vi "statusindicatorwithactivate.vi"(6 "String":string, 9 "Power":bool, 11 "Activate":bool) -> (0 "?":bool, 1 "?":bool, 2 "?":bool, 3 "?":bool, 4 "?":string)   [LabVIEW 2018, in "com.insstat.lvlib"]
uses:
  com.insstat.lvlib
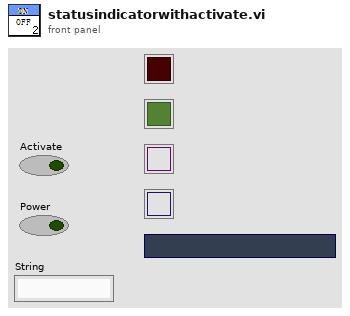
[diagram p1: front panel]
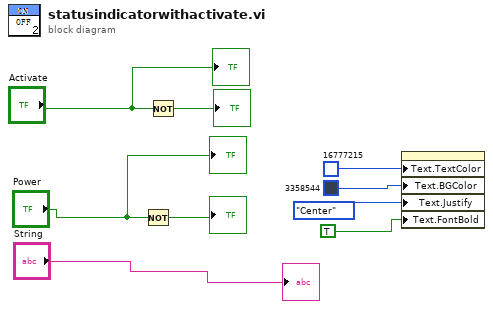
[diagram p0: block diagram]
diagram:
  n1 = Not(x="Power") -> (.not. x?=→"?":bool)
  n2 = Not(x="Activate") -> (.not. x?=→"?":bool)
  n3 = property class="Str"("Text.TextColor"=u32 16777215, "Text.BGColor"=u32 3358544, "Text.Justify"=enum16{"Left", "Center", "Right"}."Center" ("Text.Justification"), "Text.FontBold"=TRUE ("Text.Font:Bold")) -> ()  [unwired: 2 in, 2 out]
  "?" <- "Power"
  "?" <- "String"
  "?" <- "Activate"
